vi "Get Trigger Data.vi"(11 "Assembler in":refnum<class "Assembler.lvclass">) -> (2 "Trigger Data":string, 3 "Assembler out":refnum<class "Assembler.lvclass">)   [LabVIEW 2019, in "TimingDRV Engine.lvlib" / "Assembler.lvclass"]
uses:
  Assembler.lvclass
  Assembler.lvclass/Assembler.ctl
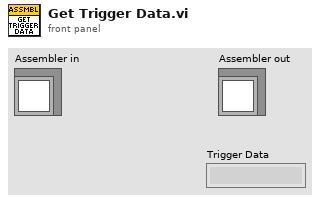
[diagram p1: front panel]
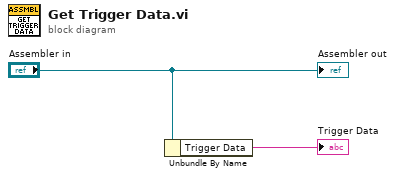
[diagram p0: block diagram]
diagram:
  n1 = Unbundle By Name("Assembler in") -> ("Trigger Data"=→"Trigger Data":string)
  "Assembler out" <- "Assembler in"
